vi "magnet without drive coil times.vi"(8 "error in (no error)":errorcluster, 9 "min time":dbl=-inf, 10 "max time":dbl=inf, 11 "display queues":T2) -> (0 "error out":errorcluster, 2 "not currently in coil veto":bool, 3 "mag no drive":T1[](array[typedef]))   [LabVIEW 2017]
uses:
  typedefs/queue cluster.ctl
  typedefs/reading1.ctl
  typedefs/reading3.ctl
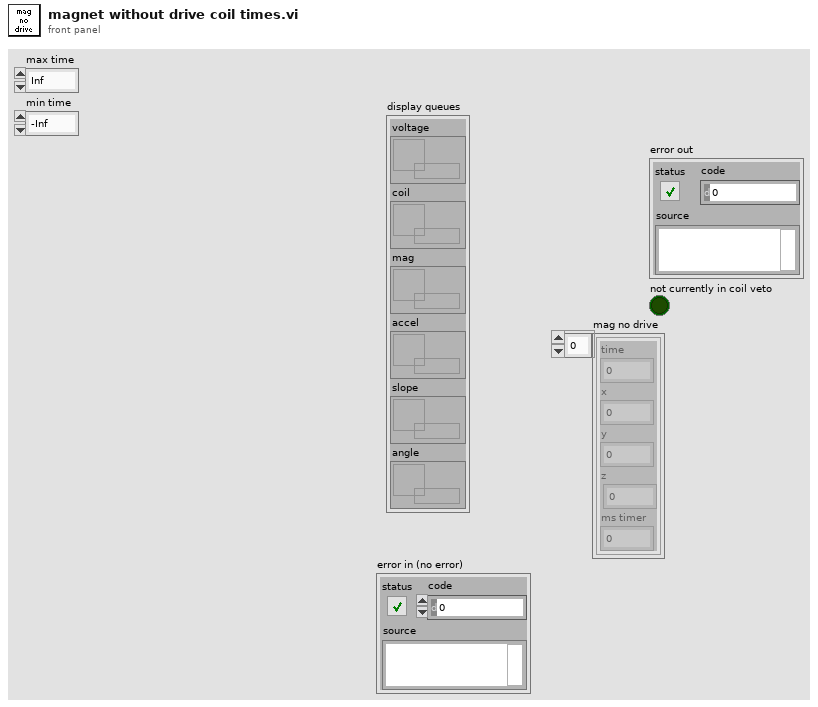
[diagram p1: front panel]
types:
  T1 = typedef "reading3.ctl" = cluster{"time":dbl, "x":dbl, "y":dbl, "z":dbl, "ms timer":u32}
  T2 = typedef "queue cluster.ctl" = cluster{"voltage":refnum<queue>, "coil":refnum<queue>, "mag":refnum<queue>, "accel":refnum<queue>, "slope":refnum<queue>, "angle":refnum<queue>}
  T3 = typedef "reading1.ctl" = cluster{"time":dbl, "x":dbl, "ms timer":u32}
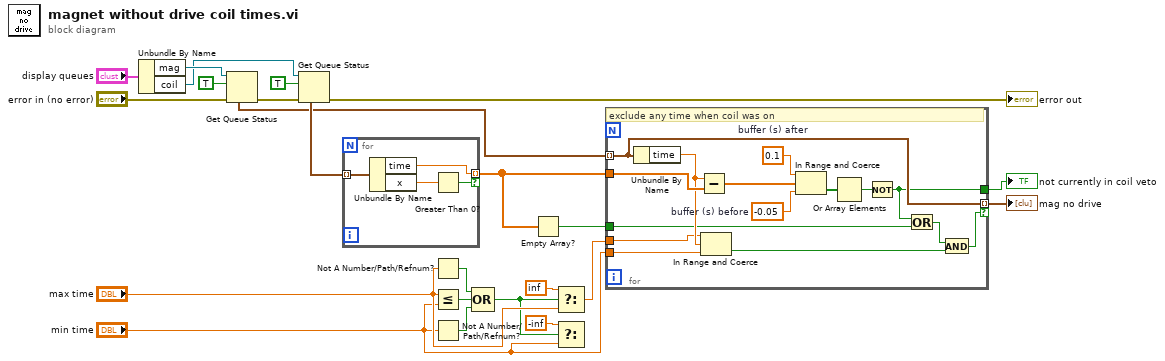
[diagram p0: block diagram]
diagram:
  n1 = Unbundle By Name("display queues") -> ("mag"=w23:refnum<queue>, "coil"=w20:refnum<queue>)
  n2 = Get Queue Status(queue=w23, return elements? (F)=TRUE, error in (no error)="error in (no error)") -> (error out=w19:errorcluster, elements=w13:T1[])  [unwired: 6 out]
  n3 = Get Queue Status(queue=w20, return elements? (F)=TRUE, error in (no error)=w19) -> (error out=→"error out":errorcluster, elements=w17:T3[])  [unwired: 6 out]
  n4 = for {
    tunnel: w17 -> [w26] mode=indexing
    tunnel: [w24] -> w11 mode=indexing if=w25
    n5 = Unbundle By Name(w26) -> ("time"=w24:dbl, "x"=w27:dbl)
    n6 = Greater Than 0?(x=w27) -> (x > 0?=w25:bool)
  }
  n7 = Not A Number/Path/Refnum?(number/path/refnum="max time") -> (NaN/Path/Refnum?=w3:bool)
  n8 = Less Or Equal?(x="max time", y="min time") -> (x <= y?=w4:bool)
  n9 = Not A Number/Path/Refnum?(number/path/refnum="min time") -> (NaN/Path/Refnum?=w2:bool)
  n10 = Compound Arithmetic op=OR(w3, w4, w2) -> (w1:bool)
  n11 = Empty Array?(array=w11) -> (empty?=w10:bool)
  n12 = Select(t=inf, s=w1, f="max time") -> (s? t:f=w8:dbl)
  n13 = Select(t=-inf, s=w1, f="min time") -> ()  [unwired: 1 out]
  n14 = for {
    tunnel: w13 -> [w42] mode=indexing
    tunnel: [w42] -> w12 mode=indexing if=w33
    tunnel: w11 -> [w41]
    tunnel: [w35] -> w14
    tunnel: w10 -> [w30]
    tunnel: w8 -> [w29]
    tunnel: "min time" -> [w28]
    w38 = -0.05  # buffer (s) before
    w39 = 0.1  # buffer (s) after
    # "exclude any time when coil was on"
    n15 = Unbundle By Name(w42) -> ("time"=w34:dbl)
    n16 = Subtract(x=w34, y=w41) -> (x-y=w40:dbl[])
    n17 = In Range and Coerce(upper limit=w29, x=w34, lower limit=w28) -> (In Range?=w32:bool)  [unwired: 1 out]
    n18 = In Range and Coerce(upper limit=w39, x=w40, lower limit=w38) -> (In Range?=w37:bool[])  [unwired: 1 out]
    n19 = Or Array Elements(Boolean array=w37) -> (logical OR=w36:bool)
    n20 = Not(x=w36) -> (.not. x?=w35:bool)
    n21 = Or(x=w35, y=w30) -> (x .or. y?=w31:bool)
    n22 = And(x=w31, y=w32) -> (x .and. y?=w33:bool)
  }
  "not currently in coil veto" <- w14
  "mag no drive" <- w12
